vi "XIPIN_ATC2_(ChipScope_Pro_-_Agilent_Trace_Core_2)_1_05_a.vi"   [LabVIEW 2017]
doc: "The Agilent Trace Core 2 (ATC2) is a customizable debug capture core that is specially designed to work with the latest generation logic analyzers from Agilent Technologies. The ATC2 core provides external Agilent logic analyzers access to internal FPGA design nets.\n------------------------------------\n<b>Need License</b> : No"
uses:
  <vilib>/rvi/XilinxIP/XIPIN_XNode/niFpgaXIPIN.xnode
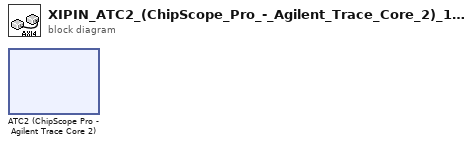
[diagram p0: block diagram]
diagram:
  n1 = xnode ("ATC2 (ChipScope Pro - Agilent Trace Core 2)")() -> ()
